vi "RD Analog Out Node Offset Amp Set.vi"(0 "handle":u64, 1 "amp":dbl, 5 "ch":i32, 7 "node":i32, 9 "vOffset":dbl, 11 "error in (no error)":errorcluster caption="错误输入（无错误）", 12 "CalArray":u8[](array[numeric])) -> (4 "handle out":u64, 6 "function return":i32, 14 "CalArray out":u8[](array[numeric]), 15 "error out":errorcluster caption="错误输出")   [LabVIEW 2018, in "InstrumentsPlayground.lvlib"]
doc: "CLIFFAPI int CliffAnalogOutNodeOffsetSet(FT_HANDLE handle, int ch, CLIFFAnalogOutNode node, double vOffset);CLIFFAPI int CliffAnalogOutNodeOffsetAmpSet(FT_HANDLE handle, int ch, CLIFFAnalogOutNode node, double vOffset,double amp);\nCLIFFAPI int CliffAnalogOutNodeOffsetAmpSet(FT_HANDLE handle, int ch, CLIFFAnalogOutNode node, double vOffset,double amp,int* CalArray);"
uses:
  InstrumentsPlayground.lvlib
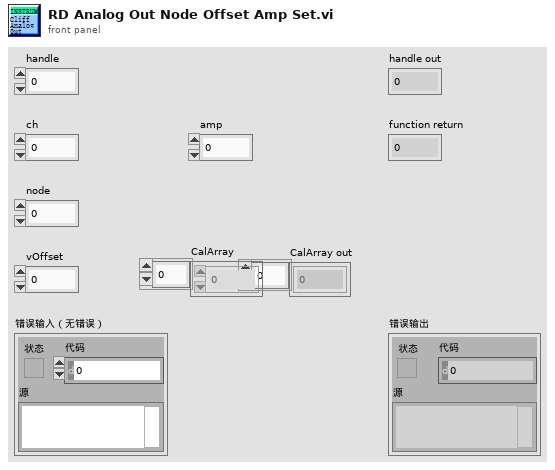
[diagram p1: front panel]
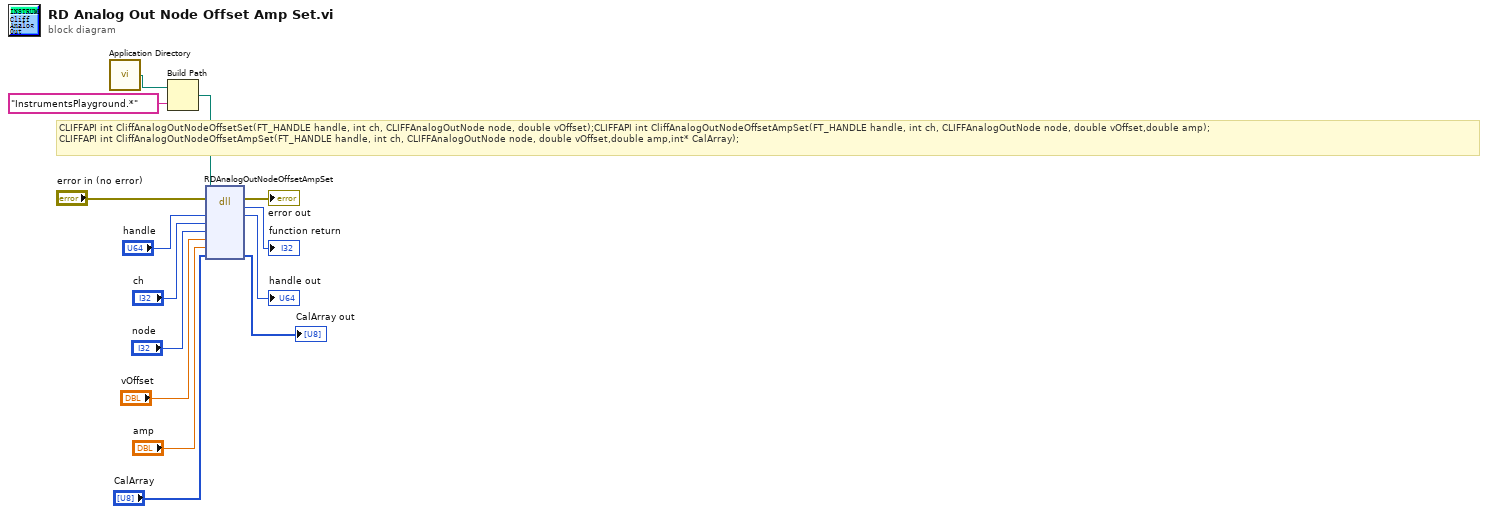
[diagram p0: block diagram]
diagram:
  # "CLIFFAPI int CliffAnalogOutNodeOffsetSet(FT_HANDLE handle, int ch, CLIFFAnalogOutNode node, double vOffset);CLIFFAPI int CliffAnalogOutNodeOffsetAmpSet(FT_HANDLE handle, int ch, CLIFFAnalogOutNode node, double vOffset,double amp);\nCLIFFAPI int CliffAnalogOutNodeOffsetAmpSet(FT_HANDLE handle, int ch, CLIFFAnalogOutNode node, double vOffset,double amp,int* CalArray);"
  n1 = call <vilib>:"Application Directory.vi"() -> ("Application Directory"=w4:path)
  n2 = Build Path(base path=w4, name or relative path="InstrumentsPlayground.*" ("名称或相对路径")) -> (appended path=w3:path)
  n3 = dll-call lib="E:/Work/YZCourse_Xtext/Cliff/API/IPLabView lib/InstrumentsPlayground.*" fn="RDAnalogOutNodeOffsetAmpSet"(path in=w3, error in="error in (no error)", "handle"="handle", "ch"="ch", "node"="node", "vOffset"="vOffset", "amp"="amp", "CalArray"="CalArray") -> (error out=→"error out":errorcluster, "返回类型"=→"function return":i32, "handle"=→"handle out":u64, "CalArray"=→"CalArray out":u8[])  [unwired: 5 in, 1 out]
